vi "Create.vi"(6 "Server Certificate File (.crt)":path, 8 "error in (no error)":errorcluster, 9 "VI Reference":refnum<vi>, 10 "Manager Address":string, 11 "CIF_UI in":refnum<class "CIF_UI.lvclass">) -> (0 "error out":errorcluster, 3 "CIF_UI out":refnum<class "CIF_UI.lvclass">)   [LabVIEW 2021, in "CIF_UI.lvclass"]
uses:
  CIF_UI.lvclass
  CIF_UI.lvclass/CIF_UI.ctl
  CIFPluginManager/CIFPluginManager/gRPC/CIF_Manager_Client_Wrapper/CIFManagerClientWrapper.lvlib
  <vilib>/gRPC/LabVIEW gRPC Library/Shared/grpcId.ctl
  <vilib>/gRPC/LabVIEW gRPC Library/grpc-lvsupport-release.lvlib
  CIFPluginManager/CIFPluginManager/gRPC/CIF_Manager_client/RPC Messages/cif_manager_PluginVersion.ctl
  CIFPluginManager/CIFPluginManager/gRPC/CIF_Manager_client/CIF_Manager_client.lvlib
  CIFPluginManager/CIFPluginManager/gRPC/CIF_Manager_client/RPC Messages/cif_plugincore_StatusData_State.ctl
  CIFPluginManager/CIFPluginManager/gRPC/CIF_Manager_client/RPC Messages/cif_plugincore_TimingStatsBasic.ctl
  CIFPluginManager/CIFPluginManager/gRPC/CIF_Manager_client/RPC Messages/cif_plugincore_TimingStatistics.ctl
  CIFPluginManager/CIFPluginManager/gRPC/CIF_Manager_client/RPC Messages/cif_plugincore_FifoStatistics.ctl
  CIFPluginManager/CIFPluginManager/gRPC/CIF_Manager_client/RPC Messages/cif_plugincore_Error.ctl
  CIFPluginManager/CIFPluginManager/gRPC/CIF_Manager_client/RPC Messages/cif_plugincore_MonitorDoubles.ctl
  CIFPluginManager/CIFPluginManager/gRPC/CIF_Manager_client/RPC Messages/cif_plugincore_MonitorU64.ctl
  CIFPluginManager/CIFPluginManager/gRPC/CIF_Manager_client/RPC Messages/cif_plugincore_MonitorI64.ctl
  CIFPluginManager/CIFPluginManager/gRPC/CIF_Manager_client/RPC Messages/cif_plugincore_StatusData.ctl
  CIFPluginManager/CIFPluginManager/gRPC/CIF_Manager_client/RPC Messages/cif_manager_PluginInfo.ctl
  Typedef/Plugin Connections.ctl
  Typedef/Plugin Connection Map.ctl
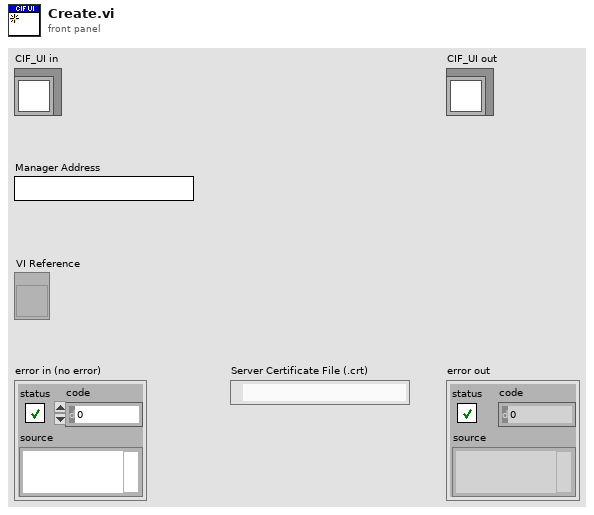
[diagram p1: front panel]
types:
  T1 = typedef "CIF_UI.lvclass/Plugin Connection Map.ctl" = map{string, T2}
  T2 = typedef "CIF_UI.lvclass/Plugin Connections.ctl" = cluster{"gRPC ID":T3, "Plugin info":T4}
  T3 = typedef "grpc-lvsupport-release.lvlib/grpcId.ctl" = u64
  T4 = typedef "CIF_Manager_client.lvlib/cif_manager_PluginInfo.ctl" = cluster{"plugin_name":string, "plugin_type":string, "grpc_port":i32, "plugin_version":T5, "status":T6}
  T5 = typedef "CIF_Manager_client.lvlib/cif_manager_PluginVersion.ctl" = cluster{"major_version":i32, "minor_version":i32, "fix_version":i32, "build_version":i32}
  T6 = typedef "CIF_Manager_client.lvlib/cif_plugincore_StatusData.ctl" = cluster{"state":T7, "timing_statistics":T8, "fifo_statistics":T10, "error":T11, "monitor_doubles":T12, "monitor_u64s":T13, "monitor_i64s":T14}
  T7 = typedef "CIF_Manager_client.lvlib/cif_plugincore_StatusData_State.ctl" = enum32{"NULL", "CREATING", "LISTENING", "RUNNING", "CLEANINGUP", "DESTROYING"}
  T8 = typedef "CIF_Manager_client.lvlib/cif_plugincore_TimingStatistics.ctl" = cluster{"period":T9, "wake_error":T9, "execute":T9, "housekeep":T9, "idle":T9}
  T9 = typedef "CIF_Manager_client.lvlib/cif_plugincore_TimingStatsBasic.ctl" = cluster{"max":i32, "min":i32}
  T10 = typedef "CIF_Manager_client.lvlib/cif_plugincore_FifoStatistics.ctl" = cluster{"from_t0":T9, "from_previous_plugin":T9, "output_error":T9}
  T11 = typedef "CIF_Manager_client.lvlib/cif_plugincore_Error.ctl" = cluster{"status":bool, "code":i32}
  T12 = typedef "CIF_Manager_client.lvlib/cif_plugincore_MonitorDoubles.ctl" = cluster{"double_1":dbl, "double_2":dbl, "double_3":dbl, "double_4":dbl}
  T13 = typedef "CIF_Manager_client.lvlib/cif_plugincore_MonitorU64.ctl" = cluster{"u64_1":u64, "u64_2":u64, "u64_3":u64, "u64_4":u64}
  T14 = typedef "CIF_Manager_client.lvlib/cif_plugincore_MonitorI64.ctl" = cluster{"i64_1":i64, "i64_2":i64, "i64_3":i64, "i64_4":i64}
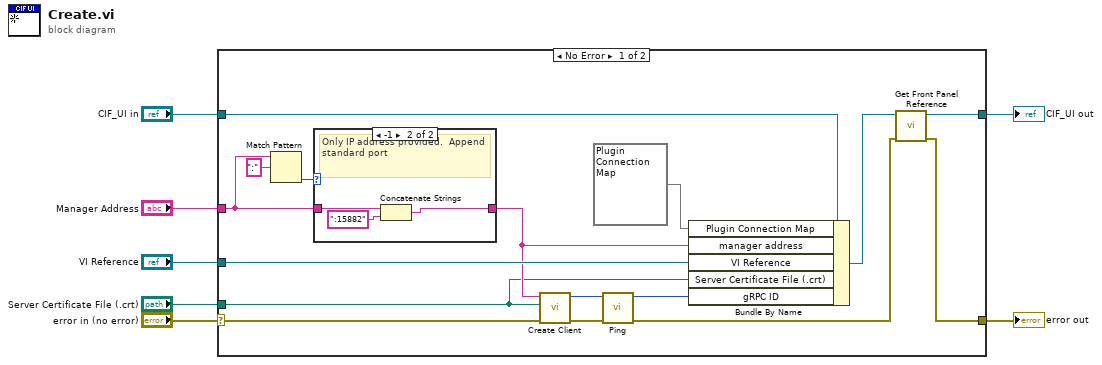
[diagram p0: block diagram]
diagram:
  n1 = case shown="No Error" "error in (no error)" {
    selector: "error in (no error)" -> [w21 w29]
    tunnel: [w20 w29] -> w6
    tunnel: [w19 w28] -> w4
    tunnel: "CIF_UI in" -> [w22 w28]
    tunnel: "Manager Address" -> [w11 _]
    tunnel: "VI Reference" -> [w23 _]
    tunnel: "Server Certificate File (.crt)" -> [w9 _]
    frame No Error {
      n2 = Match Pattern(string=w11, regular expression=":") -> (offset past match=w14:i32)  [unwired: 1 in, 3 out]
      n3 = case shown="-1" w14 {
        tunnel: w11 -> [w24 w27]
        tunnel: [w24 w26] -> w12
        frame 0, Default {
          # "Address and port provided.  Assume override and don't modify."
        }
        frame -1 {
          # "Only IP address provided.  Append standard port"
          n4 = Concatenate Strings(w27, ":15882" ("string")) -> (w26:string)
        }
      }
      n5 = call "Create Client.vi"("error in"=w21, "Server Certificate File (.crt)"=w9, "address"=w12) -> ("error out"=w18:errorcluster, "gRPC ID Out"=w15:T3)  [unwired: 7 in]
      n6 = call "Ping.vi"("error in"=w18, "gRPC ID in"=w15) -> ("error out"=w17:errorcluster, "gRPC ID out"=w10:T3)  [unwired: 8 in]
      n7 = Bundle By Name(cluster=w22, "Plugin Connection Map"=T1 {}, "manager address"=w12, "VI Reference"=w23, "Server Certificate File (.crt)"=w9, "gRPC ID"=w10) -> (w16:refnum<class "CIF_UI.lvclass">)
      n8 = call "Get Front Panel Reference.vi"("error in (no error)"=w17, "CIF_UI in"=w16) -> ("error out"=w20:errorcluster, "CIF_UI out"=w19:refnum<class "CIF_UI.lvclass">)  [unwired: 8 in]
    }
    frame Error {
    }
  }
  "error out" <- w6
  "CIF_UI out" <- w4
